vi "Increment2.vi"(8 "error in (no error)":errorcluster, 10 "Numeric":dbl, 11 "TestActor in":refnum<class "TestActor2.lvclass">) -> (0 "error out":errorcluster, 3 "TestActor out":refnum<class "TestActor2.lvclass">)   [LabVIEW 2012, in "TestActor2.lvclass"]
uses:
  TestActor2.lvclass
  <vilib>/ActorFramework/Actor/Actor.lvclass/Actor.ctl
  <vilib>/ActorFramework/Message Enqueuer/Message Enqueuer.lvclass/Message Enqueuer.ctl
  TestActor2.lvclass/TestActor2.ctl
  Increment2 Msg/Increment2 Msg.lvclass/Increment2 Msg.ctl
  <vilib>/ActorFramework/Stop Msg/Stop Msg.lvclass/Stop Msg.ctl
  <vilib>/ActorFramework/Message Enqueuer/Init from Existing Queue.vi
  <vilib>/ActorFramework/Message Enqueuer/Enqueue.vi
  <vilib>/ActorFramework/Message Enqueuer/Enqueue Critical.vi
  <vilib>/ActorFramework/Message Priority Queue/Priority Enqueue.vi
  <vilib>/ActorFramework/Message Enqueuer/Message Enqueuer.lvclass
  Increment2 Msg/Increment2 Msg.lvclass
  <vilib>/ActorFramework/Stop Msg/Stop Msg.lvclass
  <vilib>/ActorFramework/Actor/Actor.lvclass
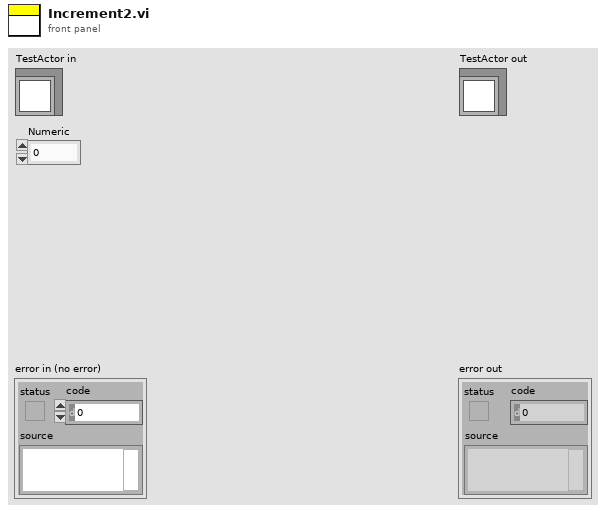
[diagram p1: front panel]
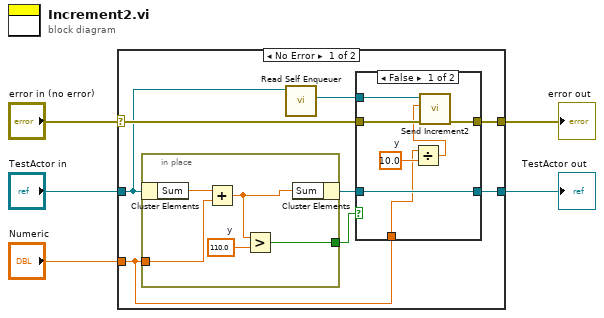
[diagram p0: block diagram]
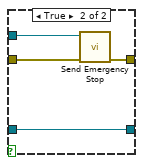
[diagram p2: hidden frame]
diagram:
  n1 = case shown="No Error" "error in (no error)" {
    selector: "error in (no error)" -> [w10 w31]
    tunnel: [w9 w31] -> w4
    tunnel: [w11 w30] -> w2
    tunnel: "TestActor in" -> [w7 w30]
    tunnel: "Numeric" -> [w8 _]
    frame No Error {
      n2 = in-place {
        in-place-border: w8 -> [w28]
        in-place-border: [w25] -> w13
        w26 = 110.0  # y
        n3 = in-place-cluster #1(w7) -> ("Sum"=w29:dbl)
        n4 = Add(x=w29, y=w28) -> (x+y=w27:dbl)
        n5 = Greater?(x=w27, y=w26) -> (0:w25:bool)
        n6 = in-place-cluster #1("Sum"=w27) -> (w12:refnum<class "TestActor2.lvclass">)
      }
      n7 = call <vilib>:"Read Self Enqueuer.vi"("Actor"=w7) -> ("Self Enqueuer"=w6:refnum<class "Message Enqueuer.lvclass">)  [unwired: 10 in]
      n8 = case shown="False" w13 {
        tunnel: w12 -> [w20 w24]
        tunnel: [w20 w24] -> w11
        tunnel: w10 -> [w19 w23]
        tunnel: [w18 w22] -> w9
        tunnel: w6 -> [w17 w21]
        tunnel: w8 -> [w15 _]
        frame False {
          w16 = 10.0  # y
          n9 = Divide(x=w15, y=w16) -> (x/y=w14:dbl)
          n10 = call "Send Increment2.vi"("error in (no error)"=w19, "Numeric"=w14, "Message Enqueuer"=w17) -> ("error out"=w18:errorcluster)  [unwired: 8 in]
        }
        frame True {
          n11 = call <vilib>:"Send Emergency Stop.vi"("error in (no error)"=w23, "Message Enqueuer"=w21) -> ("error out"=w22:errorcluster)  [unwired: 9 in]
        }
      }
    }
    frame Error {
    }
  }
  "error out" <- w4
  "TestActor out" <- w2
